vi "Check Device Status.vi"(8 "error in (no error)":errorcluster, 11 "Simple Device in":refnum<class "Simple Device.lvclass">) -> (0 "error out":errorcluster, 2 "Status":bool, 3 "Simple Device out":refnum<class "Simple Device.lvclass">)   [LabVIEW 2021, in "Simple Device.lvclass"]
uses:
  Simple Device.lvclass
  Simple Device.lvclass/Simple Device.ctl
  TALOS/TALOS_PPL.lvlibp
  Libraries/Virtual Device Simulator/DeviceSim.lvlibp/DeviceReference/Simple  Virtual Device.lvclass
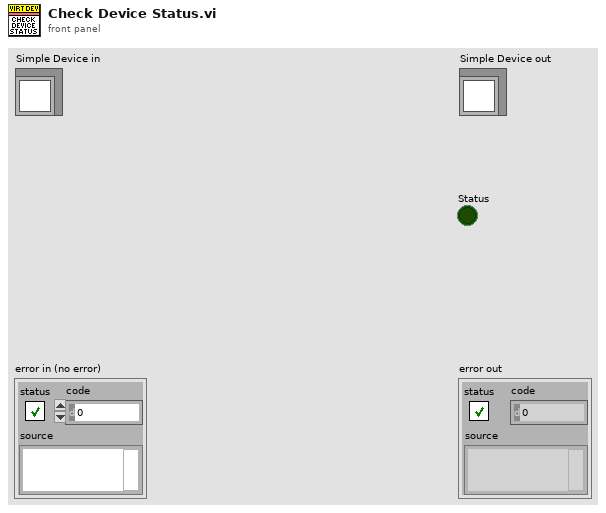
[diagram p1: front panel]
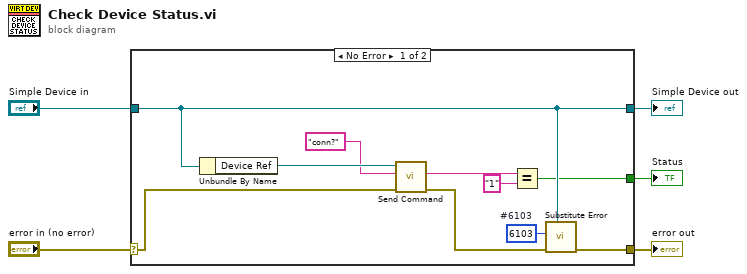
[diagram p0: block diagram]
diagram:
  n1 = case shown="No Error" "error in (no error)" {
    selector: "error in (no error)" -> [w9 w17]
    tunnel: [w14 w17] -> w4
    tunnel: [w13 w16] -> w2
    tunnel: "Simple Device in" -> [w13 w16]
    tunnel: [w12 _] -> w1
    frame No Error {
      w11 = 6103  # #6103
      n2 = Unbundle By Name(w13) -> ("Device Ref"=w10:refnum<data-value>)
      n3 = call "Send Command.vi"("error in (no error)"=w9, "Command"="conn?", "Device Ref in"=w10) -> ("error out"=w8:errorcluster, "Response"=w6:string)  [unwired: 6 in, 1 out]
      n4 = Equal?(x=w6, y="1") -> (x = y?=w12:bool)
      n5 = call "Substitute Error.vi"("LabVIEW Object"=w13, "error in (no error)"=w8, "Error Code"=w11) -> ("error out"=w14:errorcluster)  [unwired: 8 in]
    }
    frame Error {
    }
  }
  "error out" <- w4
  "Simple Device out" <- w2
  "Status" <- w1
